vi "Get Request.vi"(11 "Processing in":refnum<class "Processing.lvclass">) -> (2 "Request":refnum<class "Request.lvclass">, 3 "Processing out":refnum<class "Processing.lvclass">)   [LabVIEW 2020, in "HTTP Server.lvlib" / "Processing.lvclass"]
uses:
  Processing.lvclass
  lv-http-util/HTTP Utils/Request/Request.lvclass
  Processing.lvclass/Processing.ctl
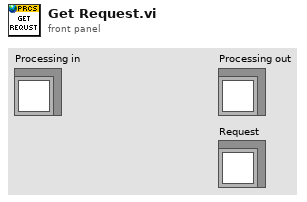
[diagram p1: front panel]
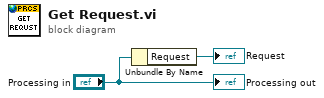
[diagram p0: block diagram]
diagram:
  n1 = Unbundle By Name("Processing in") -> ("Request"=→"Request":refnum<class "Request.lvclass">)
  "Processing out" <- "Processing in"
